vi "instance count allowed.vi"(8 "error in":errorcluster, 11 "J1939 configuration in":refnum<class "J1939 configuration.lvclass">) -> (0 "error out":errorcluster, 2 "instances allowed":i32, 3 "J1939 configuration out":refnum<class "J1939 configuration.lvclass">)   [LabVIEW 2014, in "J1939 configuration.lvclass"]
uses:
  J1939 configuration.lvclass
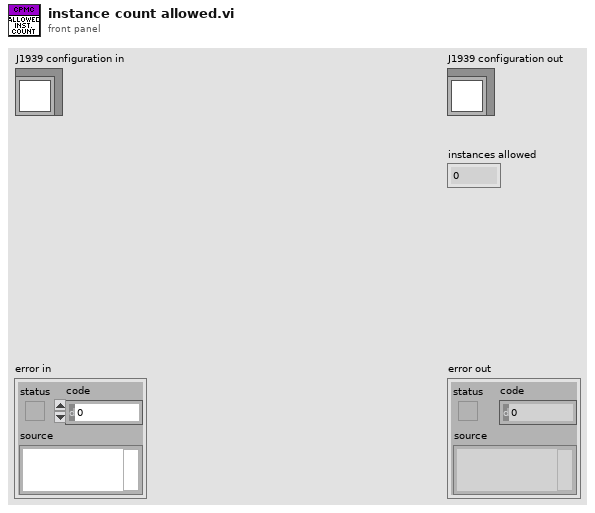
[diagram p1: front panel]
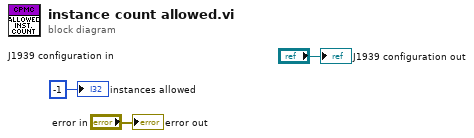
[diagram p0: block diagram]
diagram:
  "error out" <- "error in"
  "J1939 configuration out" <- "J1939 configuration in"
  "instances allowed" <- -1 ("instances allowed")
